vi "CRYData View Legend Mouse Move.vi"(8 "TotalPlot":u32, 9 "Mouse Point":T2, 10 "MCListbox Ref In":refnum<vi>) -> (0 "CellSize":T1, 1 "Position":T2, 2 "Selected Row":i32, 3 "Move State":bool, 4 "CellBG":u32)   [LabVIEW 2013]
uses:
  <vilib>/Utility/miscctls.llb/LVPositionTypeDef.ctl
  <vilib>/Utility/miscctls.llb/LVBoundsTypeDef.ctl
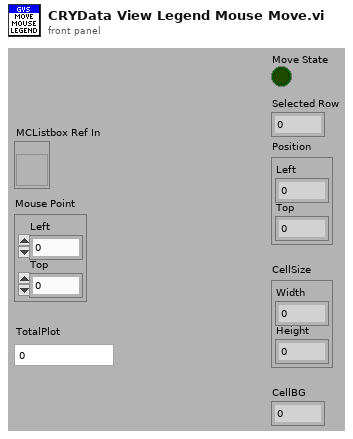
[diagram p1: front panel]
types:
  T1 = typedef "LVBoundsTypeDef.ctl" = cluster{"Width":u32, "Height":u32}
  T2 = typedef "LVPositionTypeDef.ctl" = cluster{"Left":i32, "Top":i32}
  T3 = typedef "LVRowAndColumnTypeDef.ctl" = cluster{"Row":i32, "Column":i32}
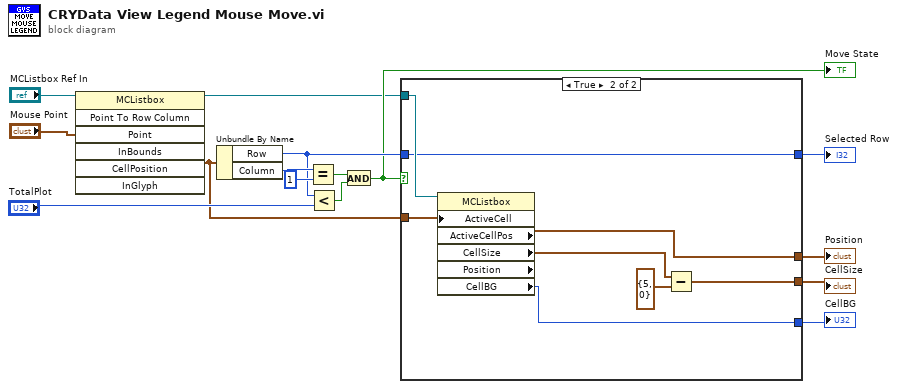
[diagram p0: block diagram]
diagram:
  n1 = invoke on="Invoke Node" class="MCListbox" method="Point To Row Column"(reference="MCListbox Ref In", "Point"="Mouse Point") -> (reference out=w7:refnum<vi>, "CellPosition"=w1:T3)  [unwired: 5 in, 5 out]
  n2 = Unbundle By Name(w1) -> ("Row"=w13:i32, "Column"=w14:i32)
  n3 = Equal?(x=w14, y=1) -> (x = y?=w12:bool)
  n4 = Less?(x=w13, y="TotalPlot") -> (x < y?=w11:bool)
  n5 = And(x=w12, y=w11) -> (x .and. y?=w10:bool)
  "Move State" <- w10
  n6 = case shown="True" w10 {
    tunnel: w1 -> [_ w23]
    tunnel: w13 -> [_ w20]
    tunnel: w7 -> [_ w21]
    tunnel: [_ w20] -> w6
    tunnel: [_ w19] -> w3
    tunnel: [_ w18] -> w4
    tunnel: [_ w17] -> w5
    frame False {
    }
    frame True {
      n7 = property on="Property Node" class="MCListbox" props=["ActiveCell", "ActiveCellPos", "CellSize", "Position", "CellBG"](reference=w21, "ActiveCell"=w23) -> ("ActiveCellPos"=w17:T2, "CellSize"=w22:T1, "CellBG"=w19:u32)  [unwired: 1 in, 3 out]
      n8 = Subtract(x=w22, y=T1 {"Width"=5, "Height"=0}) -> (x-y=w18:T1)
    }
  }
  "Position" <- w5
  "CellSize" <- w4
  "CellBG" <- w3
  "Selected Row" <- w6
